vi "utilities_checkString.vi"(8 "error in (no error)":errorcluster, 11 "String":string) -> (0 "error out":errorcluster, 3 "String out":string)   [LabVIEW 2017, in "NI_ExcelFile.lvlib"]
uses:
  <vilib>/express/express shared/NI_ExcelFile/NI_ExcelFile.lvlib
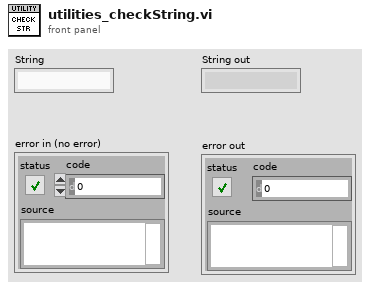
[diagram p1: front panel]
types:
  T1 = enum32{"invalid OS target", "Mac OS", "Windows 3.1", "Windows 95/NT", "Solaris 1", "Solaris 2", "HP-UX", "PowerMAX", "Linux", "Irix", "Rhapsody", "BeOS", "AIX", "OSF1", "VxWorks", "PharLap", "Carbon", "RTX", "Windows x64", "Linux x64", "Mac OS X x64"}
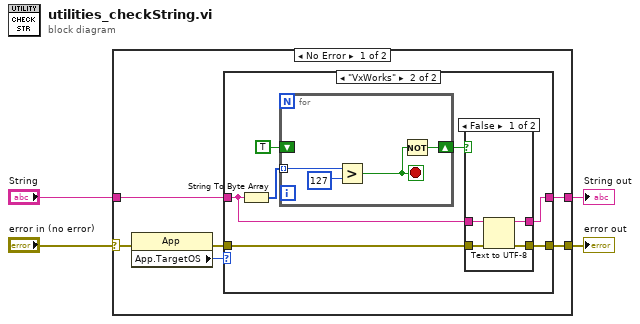
[diagram p0: block diagram]
diagram:
  n1 = case shown="No Error" "error in (no error)" {
    selector: "error in (no error)" -> [w7 w31]
    tunnel: [w10 w30] -> w4
    tunnel: "String" -> [w8 w30]
    tunnel: [w5 w31] -> w2
    frame No Error {
      n2 = property class="App"(error in=w7) -> (error out=w6:errorcluster, "App.TargetOS"=w9:T1)  [unwired: 1 in, 1 out]
      n3 = case shown="\"VxWorks\"" w9 {
        tunnel: w8 -> [w12 w15]
        tunnel: [w12 w19] -> w10
        tunnel: w6 -> [w11 w18]
        tunnel: [w11 w17] -> w5
        frame Default {
        }
        frame "VxWorks" {
          n4 = String To Byte Array(string=w15) -> (unsigned byte array=w16:u8[])
          n5 = for {
            tunnel: w16 -> [w23] mode=indexing
            shift-right: [w21] -> w14
            shift-left: TRUE -> [_]
            stop <- w20 stop-if-true
            n6 = Greater?(x=w23, y=u8 127) -> (0:w20:bool)
            n7 = Not(x=w20) -> (.not. x?=w21:bool)
          }
          n8 = case shown="False" w14 {
            tunnel: [w25 w29] -> w19
            tunnel: w15 -> [w24 w29]
            tunnel: w18 -> [w27 w28]
            tunnel: [w26 w28] -> w17
            frame False {
              n9 = Text to UTF-8(8:w27, 11:w24) -> (0:w26:errorcluster, 3:w25:string)  [unwired: 1 in]
            }
            frame True {
            }
          }
        }
      }
    }
    frame Error {
    }
  }
  "String out" <- w4
  "error out" <- w2
